vi "PH_SSAC.destructor.vi"(0 "i ref in":refnum<vi>, 5 "error in(no error)":errorcluster) -> (19 "error out":errorcluster)   [LabVIEW 2014, in "PH_SSAC.lvlib"]
doc: "This is the destructor of a class.\n\nLicense Agreement for this software:\n\nCopyright (C)\nGesellschaft für Schwerionenforschung, GSI\nPlanckstr. 1\n64291 Darmstadt\nGermany\n\nContact: D.Beck@gsi.de \n\nThis program is free software; you can redistribute it and/or modify it under the terms of the \nGNU General Public License as published by the Free Software Foundation; either version 2 of \nthe license, or (at your option) any later version.\n\nThis program is distributed in the hope that it will be useful, but WITHOUT ANY WARRANTY; \nwithout even the implied warranty of MERCHANTABILITY or FITNESS FOR A PARTICULAR PURPOSE. See the GNU General License for more details (http://www.gnu.org).\n\nGesellschaft für Schwerionenforschung, GSI\nPlanckstr. 1, 64291 Darmstadt, Germany\nFor all questions and ideas contact: M.Richter@gsi.de, H.Brand@gsi.de or D.Beck@gsi.de.\nLast update: 16-JUN-2004"
uses:
  PH_SSAC.lvlib
  PH_Img_BaseClass/PH_Img_BaseClass.lvlib
  PH_PSDBWriter/PH_PSDBWriter.lvlib
  PH_StatusHandler/PH_StatusHandler.lvlib
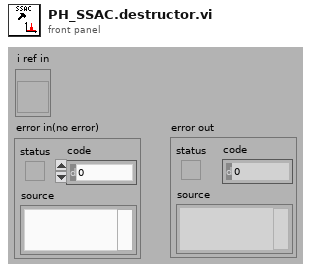
[diagram p1: front panel]
types:
  T1 = enum16{"SetAttribute", "GetAttribute", "CreateAttribute", "DestroyAttribute", "DestroyAllAtributes"}
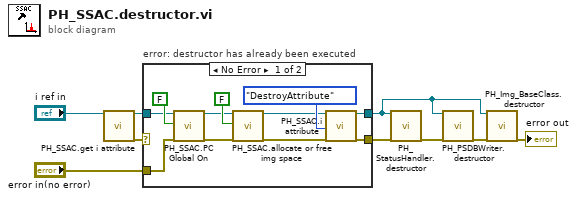
[diagram p0: block diagram]
diagram:
  n1 = call "PH_SSAC.get i attribute.vi"("i ref in"="i ref in") -> ("i ref out"=w6:refnum<vi>, "error out"=w7:errorcluster)  [unwired: 16 in, 1 out]
  n2 = case "error: destructor has already been executed" shown="No Error" w7 {
    tunnel: "error in(no error)" -> [w15 w21]
    tunnel: w6 -> [w13 w22]
    tunnel: [w19 w22] -> w1
    tunnel: [w18 w21] -> w3
    frame No Error {
      n3 = call "PH_SSAC.PC Global On.vi"("i ref in"=w13, "Global On?"=FALSE, "error in (no error)"=w15) -> ("i ref out"=w12:refnum<vi>, "error out"=w14:errorcluster)  [unwired: 15 in]
      n4 = call "PH_SSAC.allocate or free img space.vi"("i ref in"=w12, "Allocate?"=FALSE, "error in (no error)"=w14) -> ("i ref out"=w10:refnum<vi>, "error out"=w11:errorcluster)  [unwired: 15 in]
      n5 = call "PH_SSAC.i attribute.vi"("VI Refnum"=w10, "Action"=T1."DestroyAttribute", "error in (no error)"=w11) -> ("VI Refnum out"=w19:refnum<vi>, "error out"=w18:errorcluster)  [unwired: 14 in, 1 out]
    }
    frame Error {
    }
  }
  n6 = call "PH_StatusHandler.destructor.vi"("i ref in"=w1, "error in(no error)"=w3) -> ("error out"=w2:errorcluster)  [unwired: 17 in]
  n7 = call "PH_PSDBWriter.destructor.vi"("i ref in"=w1, "error in(no error)"=w2) -> ("error out"=w5:errorcluster)  [unwired: 17 in]
  n8 = call "PH_Img_BaseClass.destructor.vi"("i ref in"=w1, "error in(no error)"=w5) -> ("error out"=→"error out":errorcluster)  [unwired: 17 in]
